vi "Volt_to_board_1.vi"(8 "error in (no error)":errorcluster) -> (0 "error out":errorcluster)   [LabVIEW 2015]
doc: "This VI writes the <b>values to write</b> to the <b>addresses</b> for the specified <b>board</b>."
uses:
  <vilib>/Instr/_visa.llb/VISA Register Access Address Space.ctl
panel:
  in  "values to write":u8[](array[numeric]) format="%02d"
  in  "addresses":u32[](array[numeric]) format="%02d"
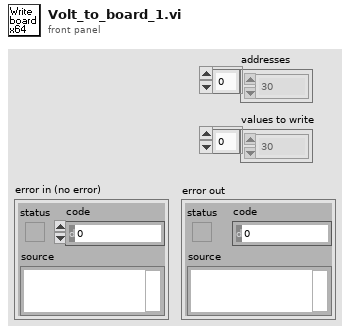
[diagram p1: front panel]
types:
  T1 = typedef "VISA Register Access Address Space.ctl" = u16
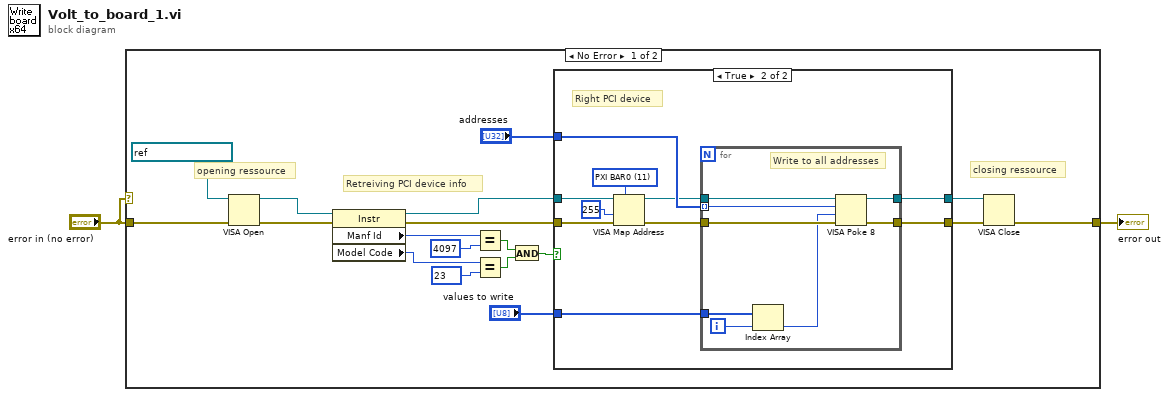
[diagram p0: block diagram]
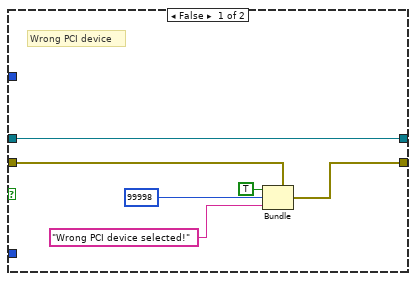
[diagram p2: hidden frame]
diagram:
  n1 = case shown="No Error" "error in (no error)" {
    tunnel: "error in (no error)" -> [w19 w45]
    tunnel: [w8 w45] -> w2
    frame No Error {
      # "closing ressource"
      # "opening ressource"
      # "Retreiving PCI device info"
      n2 = VISA Open(error in (no error)=w19, VISA resource name=refnum<visa-resource-name> "PXI4::4::INSTR" ("board")) -> (VISA resource name=w18:refnum<visa-resource-name>, error out=w17:errorcluster)  [unwired: 3 in]
      n3 = property class="Instr"(reference=w18, error in=w17) -> (reference out=w11:refnum<visa-resource-name>, error out=w7:errorcluster, "Manf Id"=w6:u16, "Model Code"=w5:u16)
      n4 = Equal?(x=w6, y=u16 4097) -> (x = y?=w14:bool)
      n5 = Equal?(x=w5, y=u16 23) -> (x = y?=w15:bool)
      n6 = And(x=w14, y=w15) -> (x .and. y?=w12:bool)
      n7 = case shown="True" w12 {
        tunnel: [w26 w36] -> w9
        tunnel: w11 -> [w26 w32]
        tunnel: w7 -> [w22 w31]
        tunnel: [w21 w35] -> w10
        tunnel: "addresses" -> [_ w34]
        tunnel: "values to write" -> [_ w27]
        frame False {
          # "Wrong PCI device"
          n8 = Bundle(cluster=w22, "status"=TRUE, "code"=99998, "source"="Wrong PCI device selected!") -> (w21:errorcluster)
        }
        frame True {
          w29 = T1 11 items=["VXI/VME A16"=1, "VXI/VME A24"=2, "VXI/VME A32"=3, "VXI/VME A64"=4, "PXI Memory Allocations"=9, "PXI Configuration"=10, "PXI BAR0"=11, "PXI BAR1"=12, "PXI BAR2"=13, "PXI BAR3"=14, "PXI BAR4"=15, "PXI BAR5"=16] ("Address Space")
          # "Right PCI device"
          n9 = VISA Map Address(7:w29, 8:w31, 9:u32 255 ("map size (0)"), 11:w32) -> (0:w30:errorcluster, 3:w33:refnum<visa-resource-name>)  [unwired: 2 in]
          n10 = for {
            tunnel: w33 -> [w41]
            tunnel: [w44] -> w36
            tunnel: w30 -> [w43]
            tunnel: [w42] -> w35
            tunnel: w34 -> [w40] mode=indexing
            tunnel: w27 -> [w38]
            i -> [w37]
            # "Write to all addresses"
            n11 = Index Array(array=w38, index=w37) -> (element=w39:u8)
            n12 = VISA Poke 8(8:w43, 9:w39, 10:w40, 11:w41) -> (0:w42:errorcluster, 3:w44:refnum<visa-resource-name>)
          }
        }
      }
      n13 = VISA Close(VISA resource name=w9, error in (no error)=w10) -> (error out=w8:errorcluster)
    }
    frame Error {
    }
  }
  "error out" <- w2
